vi "IOC shared memory initialize.vi"(10 "Shared Memory Name":string="/labview_linux_sm", 11 "Shared Memory Size (bytes)":u32=4096) -> (0 "error out":errorcluster, 2 "pointer to shared memory":u64, 3 "shared memory out":T2)   [LabVIEW 2017, in "linuxSharedMemory.lvlib"]
uses:
  linuxSharedMemory.lvlib
  <vilib>/NI/NI Linux RT IPC/Shared Memory/Controls/reference.ctl
  <vilib>/NI/NI Linux RT IPC/Shared Memory/Classes/Shared Memory/Shared Memory.lvclass
  <vilib>/NI/NI Linux RT IPC/Shared Memory/Controls/file mode.ctl
  <vilib>/NI/NI Linux RT IPC/Shared Memory/Linux RT IPC.Shared Memory.lvlib
panel:
  in  "file mode (open)":T1=enum."create/replace"
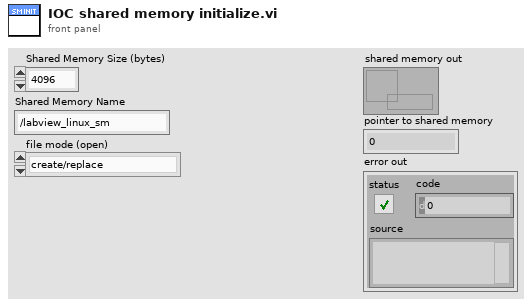
[diagram p1: front panel]
types:
  T1 = typedef "Linux RT IPC.Shared Memory.lvlib/file mode.ctl" = enum16{"open", "create/replace"}
  T2 = typedef "Linux RT IPC.Shared Memory.lvlib/reference.ctl" = refnum<data-value>
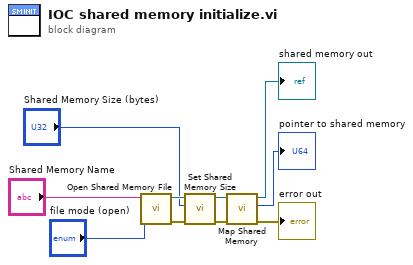
[diagram p0: block diagram]
diagram:
  n1 = call <vilib>:"Open Shared Memory File.vi"("file mode (open)"="file mode (open)", "shared memory name"="Shared Memory Name") -> ("error out"=w4:errorcluster, "shared memory out"=w5:T2)  [unwired: 8 in]
  n2 = call <vilib>:"Set Shared Memory Size.vi"("error in (no error)"=w4, "size (bytes)"="Shared Memory Size (bytes)", "shared memory in"=w5) -> ("error out"=w6:errorcluster, "shared memory out"=w7:T2)  [unwired: 7 in]
  n3 = call <vilib>:"Map Shared Memory.vi"("error in (no error)"=w6, "shared memory in"=w7) -> ("error out"=→"error out":errorcluster, "pointer to shared memory"=→"pointer to shared memory":u64, "shared memory out"=→"shared memory out":T2)  [unwired: 7 in]
